vi "Read Alice Enq.vi"(8 "error in (no error)":errorcluster, 11 "Bob in":refnum<class "Bob.lvclass">) -> (0 "error out":errorcluster, 2 "Actor Framework:Message Enqueuer":refnum<class "Message Enqueuer.lvclass">, 3 "Bob out":refnum<class "Bob.lvclass">)   [LabVIEW 2014, in "Bob.lvlib" / "Bob.lvclass"]
uses:
  Bob.lvclass
  <vilib>/ActorFramework/Message Enqueuer/Message Enqueuer.lvclass
  Bob.lvclass/Bob.ctl
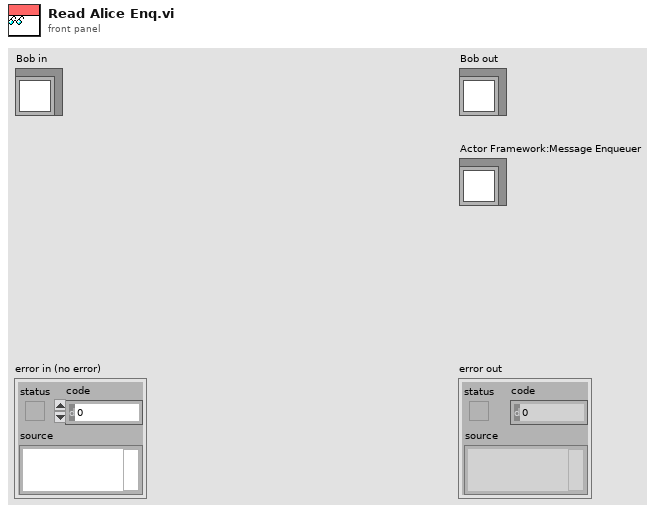
[diagram p1: front panel]
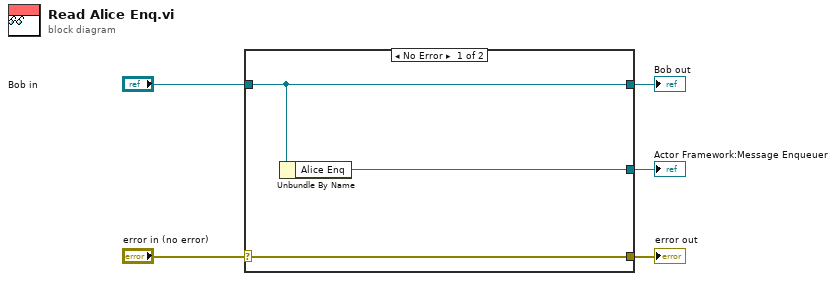
[diagram p0: block diagram]
diagram:
  n1 = case shown="No Error" "error in (no error)" {
    selector: "error in (no error)" -> [w8 w9]
    tunnel: [w8 w9] -> w4
    tunnel: [w7 w10] -> w2
    tunnel: "Bob in" -> [w7 w10]
    tunnel: [w6 _] -> w1
    frame No Error {
      n2 = Unbundle By Name(w7) -> ("Alice Enq"=w6:refnum<class "Message Enqueuer.lvclass">)
    }
    frame Error {
    }
  }
  "error out" <- w4
  "Bob out" <- w2
  "Actor Framework:Message Enqueuer" <- w1
